vi "Save for Previous Version (proj).vi"(6 "Destination Folder":path, 7 "Folder to Convert":path, 8 "error in (no error)":errorcluster, 9 "Show Front Panel?":bool, 10 "Previous Version":string(combo), 11 "vi path":path) -> (0 "error out":errorcluster)   [LabVIEW 2023]
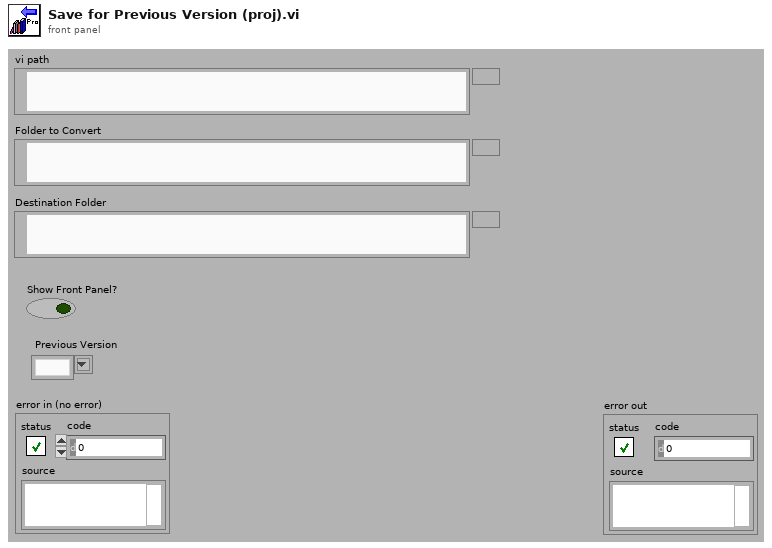
[diagram p1: front panel]
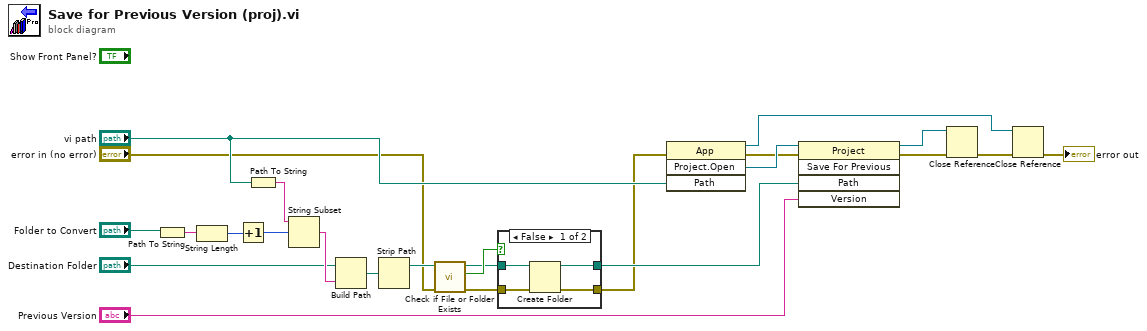
[diagram p0: block diagram]
diagram:
  n1 = Path To String(path="Folder to Convert") -> (string=w21:string)
  n2 = String Length(string=w21) -> (length=w20:i32)
  n3 = Increment(x=w20) -> (x+1=w18:i32)
  n4 = Path To String(path="vi path") -> (string=w23:string)
  n5 = String Subset(string=w23, offset (0)=w18) -> (substring=w24:string)  [unwired: 1 in]
  n6 = Build Path(base path="Destination Folder", name or relative path=w24) -> (appended path=w8:path)
  n7 = Strip Path(path=w8) -> (stripped path=w7:path)  [unwired: 1 out]
  n8 = call <vilib>:"Check if File or Folder Exists.vi"("error in (no error)"="error in (no error)", "path"=w7) -> ("error out"=w3:errorcluster, "file or folder exists?"=w6:bool, "dup path"=w5:path)  [unwired: 7 in]
  n9 = case shown="False" w6 {
    tunnel: w5 -> [w28 w30]
    tunnel: [w27 w30] -> w4
    tunnel: w3 -> [w26 w29]
    tunnel: [w25 w29] -> w1
    frame False {
      n10 = Create Folder(path (use dialog)=w28, error in=w26) -> (created path=w27:path, error out=w25:errorcluster)  [unwired: 1 in, 1 out]
    }
    frame True {
    }
  }
  n11 = invoke class="App" method="Project.Open"(error in=w1, "Path"="vi path") -> (reference out=w13:refnum<vi>, error out=w15:errorcluster, "Project:Open"=w17:refnum<vi>)  [unwired: 2 in, 1 out]
  n12 = invoke class="Project" method="Save For Previous"(reference=w17, error in=w15, "Path"=w4, "Version"="Previous Version") -> (reference out=w10:refnum<vi>, error out=w11:errorcluster)  [unwired: 1 in, 3 out]
  n13 = Close Reference(reference=w10, error in (no error)=w11) -> (error out=w9:errorcluster)
  n14 = Close Reference(reference=w13, error in (no error)=w9) -> (error out=→"error out":errorcluster)
